vi "datatype byte size.vi"(11 "Data Type":T1) -> (3 "#bytes per scalar value":i32)   [LabVIEW 2021, in "Ring Buffer Strict Accessor.lvlib"]
uses:
  Ring Buffer Strict Accessor.lvlib
  DataType.ctl
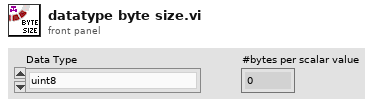
[diagram p1: front panel]
types:
  T1 = typedef "Ring Buffer Strict Accessor.lvlib/DataType.ctl" = enum16{"uint8", "uint16", "uint32", "uint64", "int8", "int16", "int32", "int64", "float", "double", "extended"}
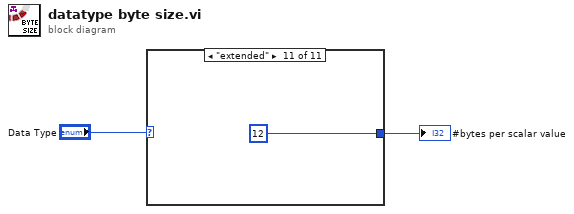
[diagram p0: block diagram]
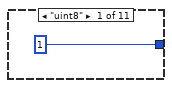
[diagram p2: hidden frame]
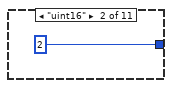
[diagram p3: hidden frame]
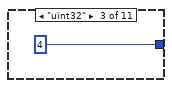
[diagram p4: hidden frame]
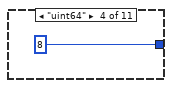
[diagram p5: hidden frame]
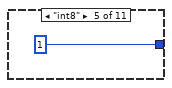
[diagram p6: hidden frame]
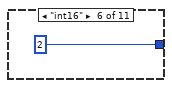
[diagram p7: hidden frame]
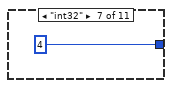
[diagram p8: hidden frame]
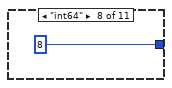
[diagram p9: hidden frame]
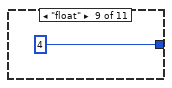
[diagram p10: hidden frame]
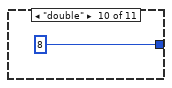
[diagram p11: hidden frame]
diagram:
  n1 = case shown="\"extended\"" "Data Type" {
    tunnel: [1 ("#bytes per value") 2 ("#bytes per value") 4 ("#bytes per value") 8 ("#bytes per value") 1 ("#bytes per value") 2 ("#bytes per value") 4 ("#bytes per value") 8 ("#bytes per value") 4 ("#bytes per value") 8 ("#bytes per value") 12 ("#bytes per value")] -> w1
    frame "uint8" {
    }
    frame "uint16" {
    }
    frame "uint32" {
    }
    frame "uint64" {
    }
    frame "int8" {
    }
    frame "int16" {
    }
    frame "int32" {
    }
    frame "int64" {
    }
    frame "float" {
    }
    frame "double" {
    }
    frame "extended" {
    }
  }
  "#bytes per scalar value" <- w1
